vi "OneTouchShotSkill.vi"(0 "object in":refnum<class "OneTouchShotSkill.lvclass">, 1 "Robot in":refnum<class "Robot.lvclass">, 5 "error in (no error)":errorcluster) -> (14 "object out":refnum<class "OneTouchShotSkill.lvclass">, 15 "Robot out":refnum<class "Robot.lvclass">, 19 "error out":errorcluster)   [LabVIEW 2023, in "OneTouchShotSkill.lvclass"]
uses:
  OneTouchShotSkill.lvclass
  Robot_class/Robot.lvclass
  OneTouchShotSkill.lvclass/OneTouchShotSkill.ctl
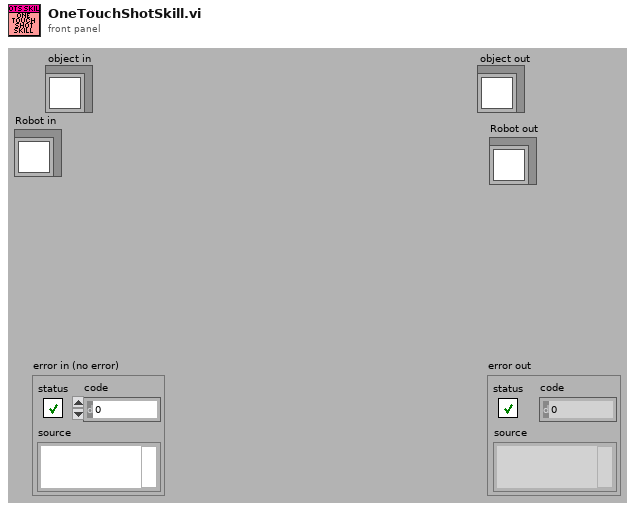
[diagram p1: front panel]
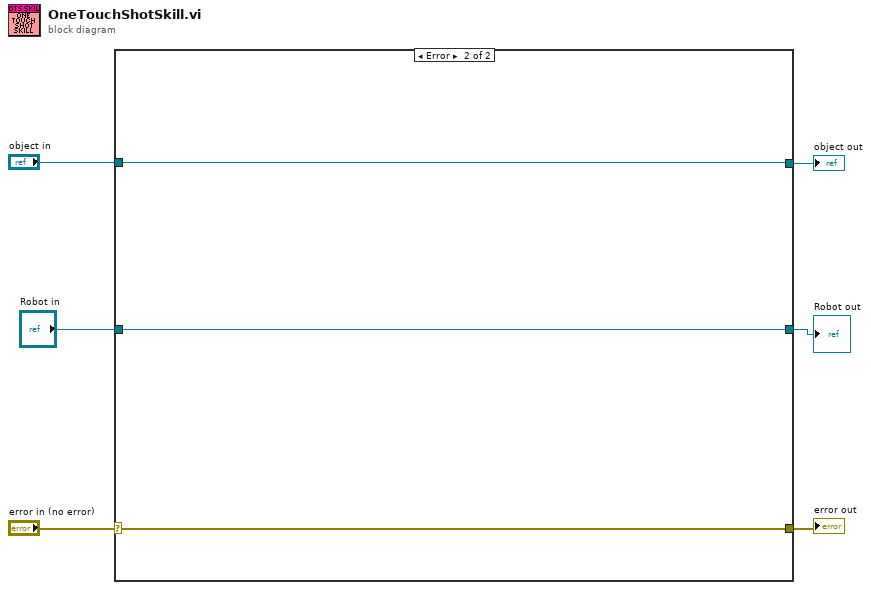
[diagram p0: block diagram]
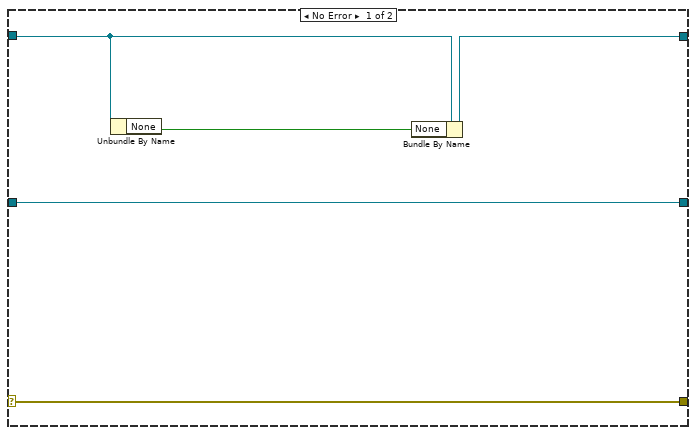
[diagram p2: hidden frame]
diagram:
  n1 = case shown="Error" "error in (no error)" {
    selector: "error in (no error)" -> [w10 w14]
    tunnel: [w10 w14] -> w5
    tunnel: [w8 w13] -> w3
    tunnel: "object in" -> [w9 w13]
    tunnel: "Robot in" -> [w7 w12]
    tunnel: [w7 w12] -> w1
    frame No Error {
      n2 = Unbundle By Name(w9) -> ("None"=w11:bool)
      n3 = Bundle By Name(cluster=w9, "None"=w11) -> (w8:refnum<class "OneTouchShotSkill.lvclass">)
    }
    frame Error {
    }
  }
  "error out" <- w5
  "object out" <- w3
  "Robot out" <- w1
